vi "sampleIndex_2_NoofSamplesinPSChans.vi"(1 "Sample Index":i32[](array[numeric])) -> (0 "No of Samples in PS Chans":i32)   [LabVIEW 2013]
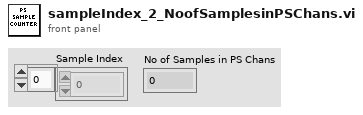
[diagram p1: front panel]
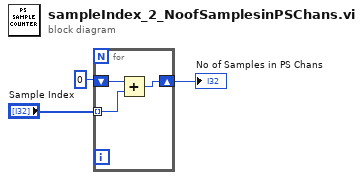
[diagram p0: block diagram]
diagram:
  n1 = for {
    tunnel: "Sample Index" -> [w4] mode=indexing
    shift-right: [w5] -> w2
    shift-left: 0 -> [w6]
    n2 = Add(x=w6, y=w4) -> (x+y=w5:i32)
  }
  "No of Samples in PS Chans" <- w2
